vi "onenote_dialogue.vi"(8 "error in (no error)":errorcluster, 11 "Image Path":path=path "C:/Users/monke/Desktop/Work/VIs to modify/ONENOTE/Sandbox/TEST.BMP") -> (0 "error out":errorcluster, 2 "Description Out":string, 3 "Image Path 2":path)   [LabVIEW 2016]
panel:
  in  "SubScript":bool
  in  "SuperScript":bool
  in  "Strikethrough":bool
  in  "Italics":bool
  in  "Bold":bool
  out "new picture":picture
  in  "Description":string="Write your description here. \nTo make text bold in OneNote, surround with <b><b/> tags.\nTo make text bold in OneNote, surround with <i><i/> tags."
  in  "Finish":bool
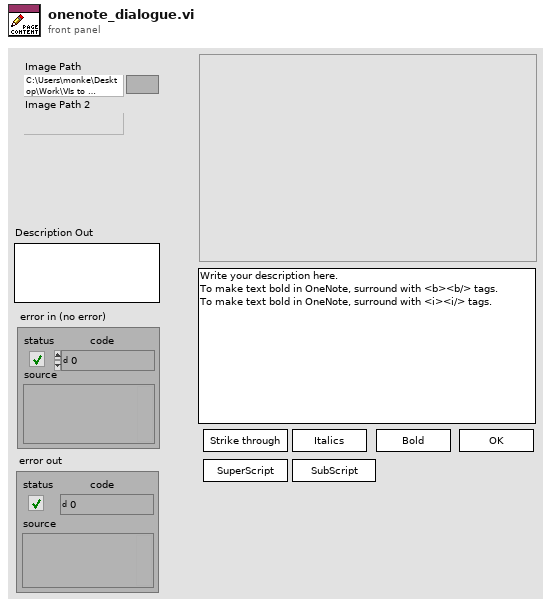
[diagram p1: front panel]
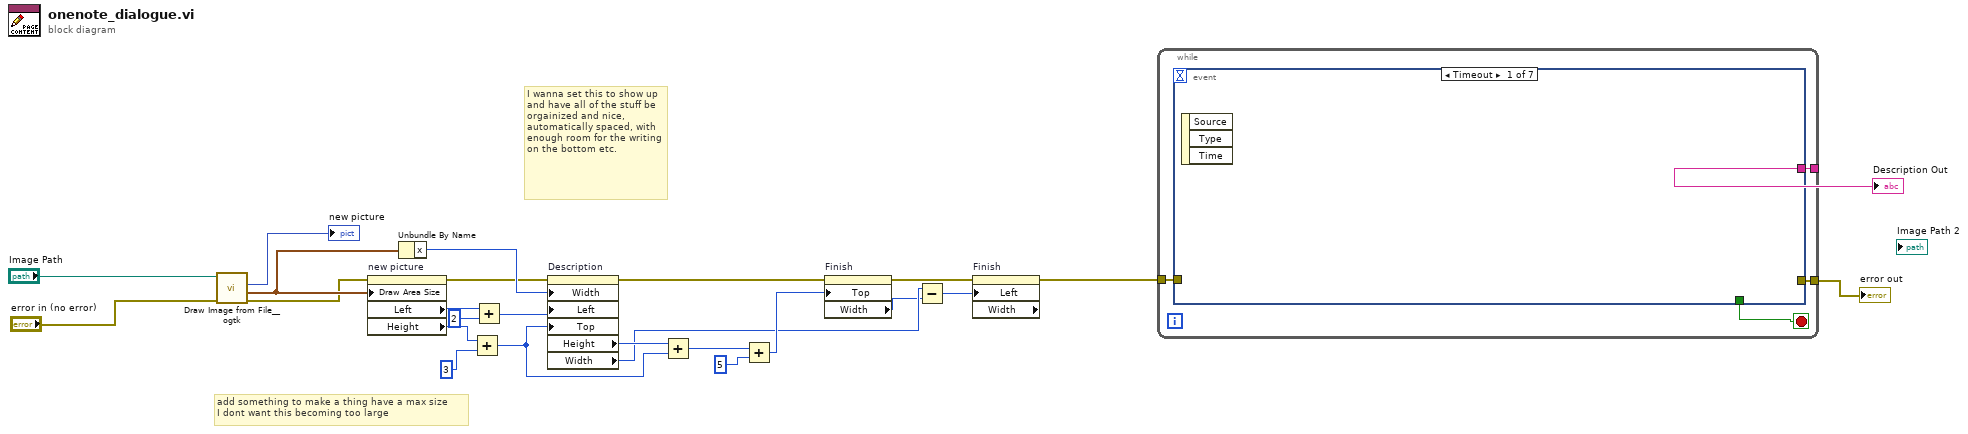
[diagram p0: block diagram]
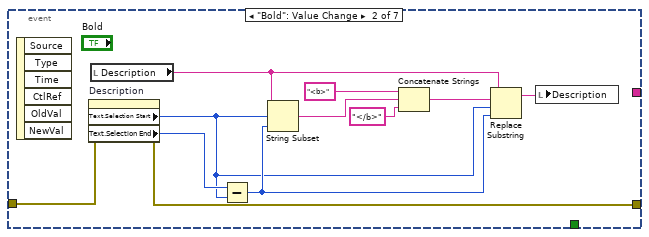
[diagram p2: hidden frame]
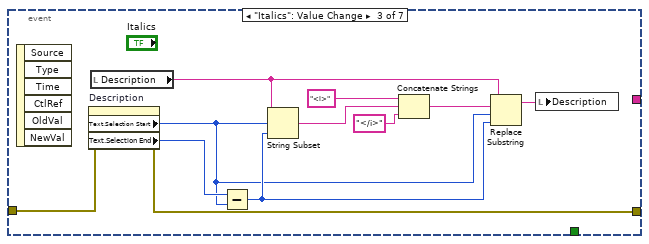
[diagram p3: hidden frame]
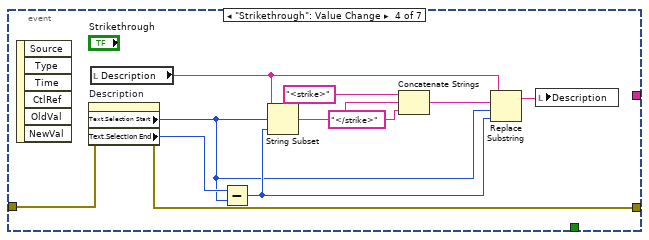
[diagram p4: hidden frame]
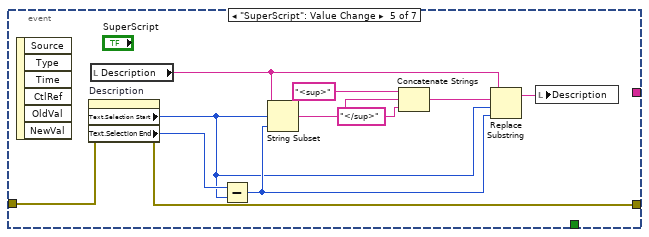
[diagram p5: hidden frame]
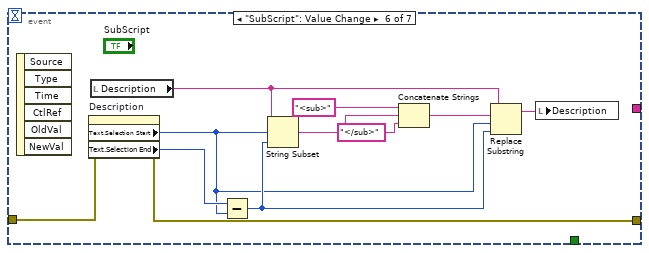
[diagram p6: hidden frame]
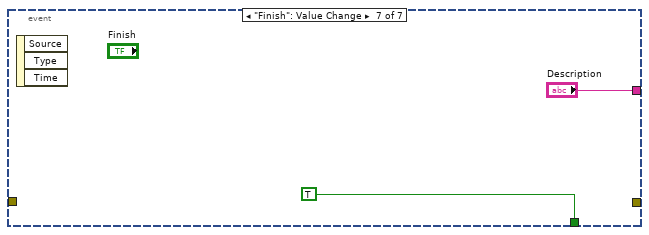
[diagram p7: hidden frame]
diagram:
  # "add something to make a thing have a max size\nI dont want this becoming too large"
  # "I wanna set this to show up and have all of the stuff be orgainized and nice, automatically spaced, with enough room for the writing on the bottom etc."
  n1 = call <userlib>:"Draw Image from File__ogtk.vi"("error in (no error)"="error in (no error)", "path to image file"="Image Path") -> ("error out"=w18:errorcluster, "image size (pixels)"=w23:cluster{"x":i16, "y":i16}, "new picture"=→"new picture":picture)  [unwired: 6 in, 1 out]
  n2 = property on="new picture" class="Pict"(error in=w18, "Draw Area Size"=w23) -> (error out=w10:errorcluster, "Left"=w20:i32, "Height"=w17:u32)  [unwired: 1 in, 1 out]
  n3 = Unbundle By Name(w23) -> ("x"=w22:i16)
  n4 = Add(x=w17, y=u32 3) -> (x+y=w12:u32)
  n5 = Add(x=w20, y=2) -> (x+y=w19:i32)
  n6 = property on="Description" class="Str"(error in=w10, "Width"=w22, "Left"=w19, "Top"=w12) -> (error out=w9:errorcluster, "Height"=w13:u32, "Width"=w7:u32)  [unwired: 1 in, 1 out]
  n7 = Add(x=w13, y=w12) -> (x+y=w11:u32)
  n8 = Add(x=w11, y=u32 5) -> (x+y=w14:u32)
  n9 = property on="Finish" class="Bool"(error in=w9, "Top"=w14) -> (error out=w8:errorcluster, "Width"=w6:u32)  [unwired: 1 in, 1 out]
  n10 = Subtract(x=w7, y=w6) -> (x-y=w5:u32)
  n11 = property on="Finish" class="Bool" props=["Left", "Width"](error in=w8, "Left"=w5) -> (error out=w1:errorcluster)  [unwired: 1 in, 2 out]
  n12 = while {
    tunnel: [w28] -> w4
    tunnel: [w27] -> w2
    tunnel: w1 -> [w26]
    stop <- w29 stop-if-true
    n13 = event shown="[0] Timeout" {
      selector: _ -> [_ _ _ _ _ _ _]
      dyn-events: _ -> [_ _ _ _ _ _ _]
      timeout: _ -> [_ _ _ _ _ _ _]
      tunnel: [_ _ _ _ _ _ TRUE] -> w29
      tunnel: [_ _ _ _ _ _ "Description"] -> w28
      tunnel: [_ w34 w45 w56 w67 w78 _] -> w27
      tunnel: w26 -> [_ w33 w44 w55 w66 w77 _]
      event Timeout {
        n14 = event-data() -> ()  [unwired: 1 in, 3 out]
      }
      event "Bold": Value Change {
        n15 = event-data() -> ()  [unwired: 1 in, 6 out]
        n16 = property on="Description" class="Str"(error in=w33) -> (error out=w34:errorcluster, "Text.Selection Start"=w30:u32, "Text.Selection End"=w40:u32)  [unwired: 1 in, 1 out]
        n17 = local read "Description"() -> (w31:string)
        n18 = Subtract(x=w40, y=w30) -> (x-y=w38:u32)
        n19 = String Subset(string=w31, offset (0)=w30, length (rest)=w38) -> (substring=w36:string)
        n20 = Concatenate Strings("<b>" ("string"), w36, "</b>" ("string")) -> (w39:string)
        n21 = Replace Substring(2:w38, 3:w30, 4:w39, 5:w31) -> (1:w35:string)  [unwired: 1 out]
        n22 = local write "Description"(w35) -> ()
      }
      event "Italics": Value Change {
        n23 = event-data() -> ()  [unwired: 1 in, 6 out]
        n24 = property on="Description" class="Str"(error in=w44) -> (error out=w45:errorcluster, "Text.Selection Start"=w41:u32, "Text.Selection End"=w51:u32)  [unwired: 1 in, 1 out]
        n25 = local read "Description"() -> (w42:string)
        n26 = Subtract(x=w51, y=w41) -> (x-y=w49:u32)
        n27 = String Subset(string=w42, offset (0)=w41, length (rest)=w49) -> (substring=w47:string)
        n28 = Concatenate Strings("<i>" ("string"), w47, "</i>" ("string")) -> (w50:string)
        n29 = Replace Substring(2:w49, 3:w41, 4:w50, 5:w42) -> (1:w46:string)  [unwired: 1 out]
        n30 = local write "Description"(w46) -> ()
      }
      event "Strikethrough": Value Change {
        n31 = event-data() -> ()  [unwired: 1 in, 6 out]
        n32 = property on="Description" class="Str"(error in=w55) -> (error out=w56:errorcluster, "Text.Selection Start"=w52:u32, "Text.Selection End"=w62:u32)  [unwired: 1 in, 1 out]
        n33 = local read "Description"() -> (w53:string)
        n34 = Subtract(x=w62, y=w52) -> (x-y=w60:u32)
        n35 = String Subset(string=w53, offset (0)=w52, length (rest)=w60) -> (substring=w58:string)
        n36 = Concatenate Strings("<strike>" ("string"), w58, "</strike>" ("string")) -> (w61:string)
        n37 = Replace Substring(2:w60, 3:w52, 4:w61, 5:w53) -> (1:w57:string)  [unwired: 1 out]
        n38 = local write "Description"(w57) -> ()
      }
      event "SuperScript": Value Change {
        n39 = event-data() -> ()  [unwired: 1 in, 6 out]
        n40 = property on="Description" class="Str"(error in=w66) -> (error out=w67:errorcluster, "Text.Selection Start"=w63:u32, "Text.Selection End"=w73:u32)  [unwired: 1 in, 1 out]
        n41 = local read "Description"() -> (w64:string)
        n42 = Subtract(x=w73, y=w63) -> (x-y=w71:u32)
        n43 = String Subset(string=w64, offset (0)=w63, length (rest)=w71) -> (substring=w69:string)
        n44 = Concatenate Strings("<sup>" ("string"), w69, "</sup>" ("string")) -> (w72:string)
        n45 = Replace Substring(2:w71, 3:w63, 4:w72, 5:w64) -> (1:w68:string)  [unwired: 1 out]
        n46 = local write "Description"(w68) -> ()
      }
      event "SubScript": Value Change {
        n47 = event-data() -> ()  [unwired: 1 in, 6 out]
        n48 = property on="Description" class="Str"(error in=w77) -> (error out=w78:errorcluster, "Text.Selection Start"=w74:u32, "Text.Selection End"=w84:u32)  [unwired: 1 in, 1 out]
        n49 = local read "Description"() -> (w75:string)
        n50 = Subtract(x=w84, y=w74) -> (x-y=w82:u32)
        n51 = String Subset(string=w75, offset (0)=w74, length (rest)=w82) -> (substring=w80:string)
        n52 = Concatenate Strings("<sub>" ("string"), w80, "</sub>" ("string")) -> (w83:string)
        n53 = Replace Substring(2:w82, 3:w74, 4:w83, 5:w75) -> (1:w79:string)  [unwired: 1 out]
        n54 = local write "Description"(w79) -> ()
      }
      event "Finish": Value Change {
        n55 = event-data() -> ()  [unwired: 1 in, 3 out]
      }
    }
  }
  "error out" <- w2
  "Description Out" <- w4
